vi "Remove Action Queue Items.vi"(8 "error in (no error)":errorcluster, 11 "Action":T1=enum."Loop Set Bleed-Fuel-ECS Cntrls") -> (0 "error out":errorcluster)   [LabVIEW 2018, in "Outputs.lvlib"]
uses:
  Outputs.lvlib
  Private Controls/Module Action.ctl
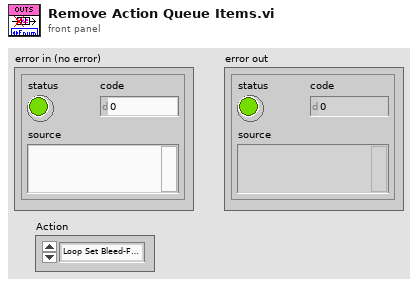
[diagram p1: front panel]
types:
  T1 = typedef "RT - Instrument IO.lvlib/Module Action.ctl" = enum16{"Init", "Error", "StartStop Acquisition", "Write 02-06-9265 Vals (AO)", "Write 00-04-9265 Vals (AO)", "Write 02-00-9485 Vals (DO)", "Write 02-01-9485 Vals (DO)", "Set APU&ECU Cntrls", "Set Bleed-Fuel-ECS Cntrls", "Loop Set Bleed-Fuel-ECS Cntrls", "Set ECS Demnd Cluster", "Set Fuel Pres Regltr", "Set Overspeed Thresholds", "Write Single 02-00-9485 Chann", "Write Single 02-01-9485 Chann", "Write Single 00-04-9265 Chann", "Set Sample Rate", "ESTOP"}
  T2 = typedef "RT - Instrument IO.lvlib/Module Data.ctl" = cluster{"Data":variant, "Action":T3}
  T3 = typedef "RT - Instrument IO.lvlib/Module Action.ctl" = enum16{"Init", "Error", "StartStop Acquisition", "Write 02-06-9265 Vals (AO)", "Write 00-04-9265 Vals (AO)", "Write 02-00-9485 Vals (DO)", "Write 02-01-9485 Vals (DO)", "Set APU&ECU Cntrls", "Set Bleed-Fuel-ECS Cntrls", "Set ECS Demnd Cluster", "Set Fuel Pres Regltr", "Write Single 02-00-9485 Chann", "Write Single 02-01-9485 Chann", "Write Single 00-04-9265 Chann", "Set Sample Rate", "ESTOP"}
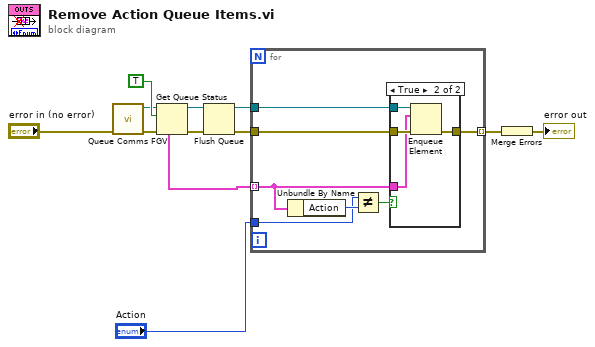
[diagram p0: block diagram]
diagram:
  n1 = call "Queue Comms FGV.vi"("error in (no error)"="error in (no error)") -> ("error out"=w2:errorcluster, "Queue out"=w1:refnum<queue>)  [unwired: 9 in]
  n2 = Get Queue Status(queue=w1, return elements? (F)=TRUE, error in (no error)=w2) -> (queue out=w6:refnum<queue>, error out=w5:errorcluster, elements=w4:T2[])  [unwired: 5 out]
  n3 = Flush Queue(queue=w6, error in (no error)=w5) -> (queue out=w8:refnum<queue>, error out=w9:errorcluster)  [unwired: 1 out]
  n4 = for {
    tunnel: w4 -> [w16] mode=indexing
    tunnel: "Action" -> [w17]
    tunnel: w8 -> [w13]
    tunnel: w9 -> [w15]
    tunnel: [w14] -> w10 mode=indexing
    n5 = Unbundle By Name(w16) -> ("Action"=w19:T3)
    n6 = Not Equal?(x=w17, y=w19) -> (x != y?=w18:bool)
    n7 = case shown="True" w18 {
      tunnel: w16 -> [_ w23]
      tunnel: w15 -> [w20 w24]
      tunnel: [w20 w22] -> w14
      tunnel: w13 -> [_ w21]
      frame False {
      }
      frame True {
        n8 = Enqueue Element(queue=w21, element=w23, error in (no error)=w24) -> (error out=w22:errorcluster)  [unwired: 1 in, 2 out]
      }
    }
  }
  n9 = Merge Errors(w10) -> (→"error out":errorcluster)
